vi "Process Raw CAN TDMS into Usable TDMS.vi"() -> ()   [LabVIEW 2014]
uses:
  <vilib>/RioEmbeddedCAN/RioEmbeddedCAN.llb/CANFrameControl.ctl
  8byte to 4 2byte.vi
  TDMS Timestamp and Data.vi
  TDMS Timestamp and Data Double.vi
  BMS/Scale Cell Voltage.vi
  BMS/Scale Cell Temp.vi
panel:
  out "error out":errorcluster
  in  "Destination":path
  in  "Source":path
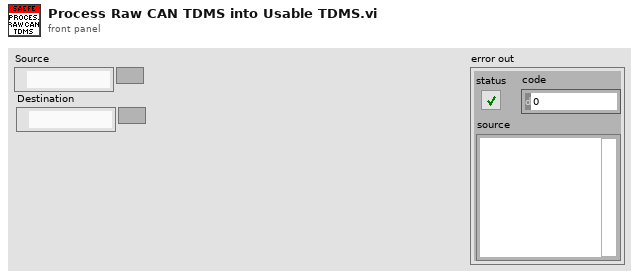
[diagram p1: front panel]
types:
  T1 = enum16{"open", "open or create", "create or replace", "create", "open (read-only)"}
  T2 = typedef "CANFrameControl.ctl" = cluster{"identifier":u32, "extended?":bool, "type":u8, "payload":u8[]}
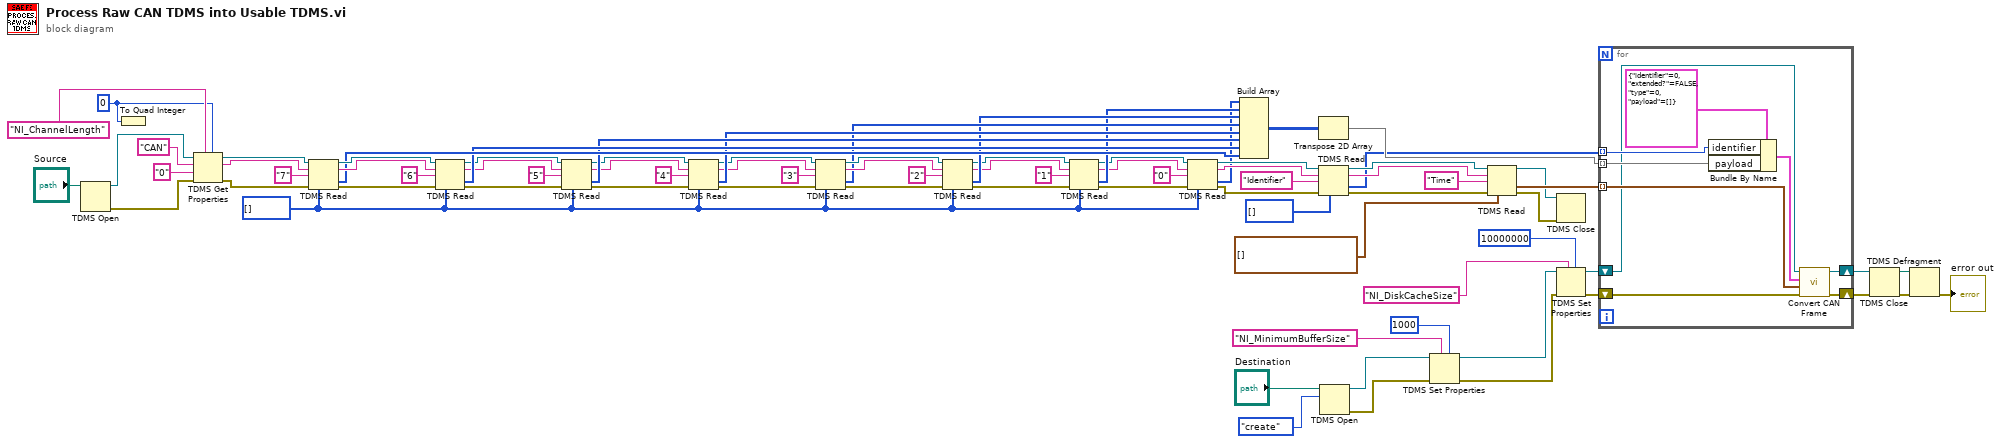
[diagram p0: block diagram]
diagram:
  w8 = u8[] []
  w75 = u64 0 ("data type")
  n1 = TDMS Open(11:"Source") -> (0:w80:errorcluster, 3:w81:refnum<k34>)  [unwired: 6 in]
  n2 = To Quad Integer(1:w75) -> ()  [unwired: 1 out]
  n3 = TDMS Get Properties(5:w75, 7:"NI_ChannelLength" ("property name"), 8:w80, 9:"0" ("channel name"), 10:"CAN" ("group name"), 11:w81) -> (0:w73:errorcluster, 2:w72:string, 3:w74:refnum<k34>)  [unwired: 3 out]
  n4 = TDMS Read(0:w74, 5:w72, 7:"7" ("channel name(s) in"), 11:w73, 12:w8) -> (4:w70:refnum<k34>, 6:w68:string, 10:w66:u8[], 15:w69:errorcluster)  [unwired: 3 in, 2 out]
  n5 = TDMS Read(0:w70, 5:w68, 7:"6" ("channel name(s) in"), 11:w69, 12:w8) -> (4:w64:refnum<k34>, 6:w62:string, 10:w65:u8[], 15:w63:errorcluster)  [unwired: 3 in, 2 out]
  n6 = TDMS Read(0:w64, 5:w62, 7:"5" ("channel name(s) in"), 11:w63, 12:w8) -> (4:w59:refnum<k34>, 6:w58:string, 10:w60:u8[], 15:w56:errorcluster)  [unwired: 3 in, 2 out]
  n7 = TDMS Read(0:w59, 5:w58, 7:"4" ("channel name(s) in"), 11:w56, 12:w8) -> (4:w54:refnum<k34>, 6:w52:string, 10:w55:u8[], 15:w53:errorcluster)  [unwired: 3 in, 2 out]
  n8 = TDMS Read(0:w54, 5:w52, 7:"3" ("channel name(s) in"), 11:w53, 12:w8) -> (4:w50:refnum<k34>, 6:w48:string, 10:w45:u8[], 15:w49:errorcluster)  [unwired: 3 in, 2 out]
  n9 = TDMS Read(0:w50, 5:w48, 7:"2" ("channel name(s) in"), 11:w49, 12:w8) -> (4:w10:refnum<k34>, 6:w4:string, 10:w44:u8[], 15:w9:errorcluster)  [unwired: 3 in, 2 out]
  n10 = TDMS Read(0:w10, 5:w4, 7:"1" ("channel name(s) in"), 11:w9, 12:w8) -> (4:w3:refnum<k34>, 6:w1:string, 10:w7:u8[], 15:w2:errorcluster)  [unwired: 3 in, 2 out]
  n11 = TDMS Read(0:w3, 5:w1, 7:"0" ("channel name(s) in"), 11:w2, 12:w8) -> (4:w43:refnum<k34>, 6:w41:string, 10:w6:u8[], 15:w42:errorcluster)  [unwired: 3 in, 2 out]
  n12 = Build Array(w6, w7, w44, w45, w55, w60, w65, w66) -> (w33:u8[][])
  n13 = Transpose 2D Array(2D array=w33) -> (transposed array=w32:u8[][])
  n14 = TDMS Read(0:w43, 5:w41, 7:"Identifier" ("channel name(s) in"), 11:w42, 12:u32[] []) -> (4:w38:refnum<k34>, 6:w36:string, 10:w30:u32[], 15:w37:errorcluster)  [unwired: 3 in, 2 out]
  n15 = TDMS Open(10:T1."create" ("operation (0:open)"), 11:"Destination") -> (0:w26:errorcluster, 3:w27:refnum<k34>)  [unwired: 5 in]
  n16 = TDMS Set Properties(5:u32 1000, 7:"NI_MinimumBufferSize", 8:w26, 11:w27) -> (0:w22:errorcluster, 3:w23:refnum<k34>)  [unwired: 2 in, 2 out]
  n17 = TDMS Read(0:w38, 5:w36, 7:"Time" ("channel name(s) in"), 11:w37, 12:timestamp[] []) -> (4:w12:refnum<k34>, 10:w31:timestamp[], 15:w11:errorcluster)  [unwired: 3 in, 3 out]
  n18 = TDMS Close(8:w11, 11:w12) -> ()  [unwired: 2 out]
  n19 = TDMS Set Properties(5:u32 10000000, 7:"NI_DiskCacheSize", 8:w22, 11:w23) -> (0:w18:errorcluster, 3:w19:refnum<k34>)  [unwired: 2 in, 2 out]
  n20 = for {
    tunnel: w32 -> [w87] mode=indexing
    tunnel: w31 -> [w88] mode=indexing
    tunnel: w30 -> [w86] mode=indexing
    shift-right: [w82] -> w16
    shift-left: w19 -> [w85]
    shift-right: [w83] -> w17
    shift-left: w18 -> [w84]
    n21 = Bundle By Name(cluster=T2 {"identifier"=0, "extended?"=FALSE, "type"=0, "payload"=[]} ("CAN frame"), "identifier"=w86, "payload"=w87) -> (w89:T2)
    n22 = call "Convert CAN Frame.vi"("error in (no error)"=w84, "timestamp"=w88, "CAN frame"=w89, "tdms file"=w85) -> ("error out"=w83:errorcluster, "tdms file out"=w82:refnum<k34>)  [unwired: 6 in]
  }
  n23 = TDMS Close(8:w17, 11:w16) -> (0:w14:errorcluster, 3:w15:path)
  n24 = TDMS Defragment(4:w14, 7:w15) -> (0:→"error out":errorcluster)
